vi "Extract Data.vi"(6 "Default body text":T1 {"Body Text Spec"."Alignment" items=["left", "center", "right"]}, 7 "Type":enum16{"VI", "Library"}(ring), 8 "error in":errorcluster, 11 "Value":variant) -> (0 "error out":errorcluster, 3 "Data":T4={"Text Visible?"=FALSE, "Text Opacity"=0, "Templ Visible?"=FALSE, "Templ Opacity"=0, "Relative Path from 1 to 2"=path "", "Image"=bytes[0], "All User Layers"=[], "Body Text"={"Line 1 text"="", "Line 2 text"="", "Line 3 text"="", "Line 4 text"="", "Line 1 color"=0, "Line 2 color"=0, "Line 3 color"=0, "Line 4 color"=0, "Body Text Spec"={"Font"="", "Alignment"=0, "Size"=3}, "Center text vertically"=FALSE, "Capitalize Text"=FALSE}} {"Body Text"."Body Text Spec"."Alignment" items=["left", "center", "right"]})   [LabVIEW 2012, in "lv_icon.lvlib"]
doc: "Extract the binary data of a LabVIEW Icon."
uses:
  <vilib>/LabVIEW Icon API/lv_icon/lv_icon.lvlib
  <vilib>/LabVIEW Icon API/lv_icon/Controls/LabVIEW Icon Stored Information.ctl
  <vilib>/LabVIEW Icon API/lv_icon/Classes/Layer/Layer.lvclass
  <vilib>/LabVIEW Icon API/lv_icon/Controls/BodyText.ctl
  <vilib>/LabVIEW Icon API/lv_icon/Controls/Font.ctl
  <vilib>/LabVIEW Icon API/lv_icon/Controls/Alignment.ctl
  <vilib>/picture/picture.llb/imagedata.ctl
  <vilib>/LabVIEW Icon API/lv_icon/Controls/LayerType.ctl
  <vilib>/LabVIEW Icon API/lv_icon/Classes/Load_Unload/Load & Unload.lvclass
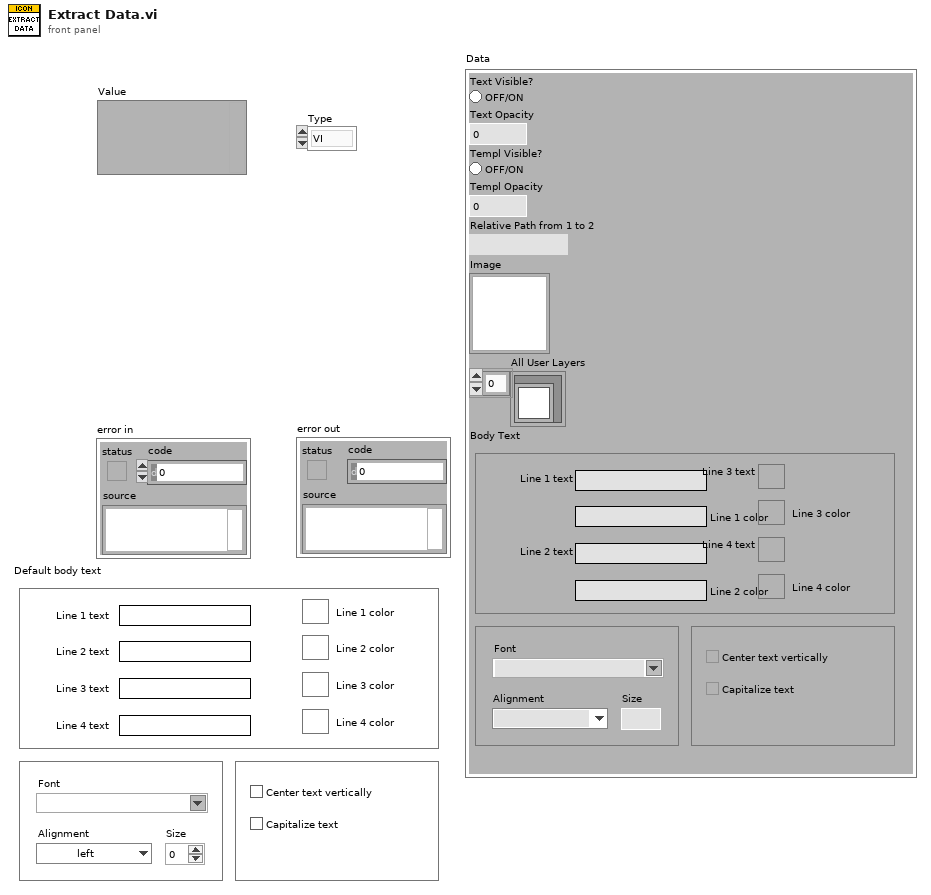
[diagram p1: front panel]
types:
  T1 = typedef "BodyText.ctl" = cluster{"Line 1 text":string, "Line 2 text":string, "Line 3 text":string, "Line 4 text":string, "Line 1 color":u32, "Line 2 color":u32, "Line 3 color":u32, "Line 4 color":u32, "Body Text Spec":cluster{"Font":T2, "Alignment":T3, "Size":u8}, "Center text vertically":bool, "Capitalize Text":bool}
  T2 = typedef "Font.ctl" = string
  T3 = typedef "Alignment.ctl" = u16
  T4 = typedef "LabVIEW Icon Stored Information.ctl" = cluster{"Text Visible?":bool, "Text Opacity":u8, "Templ Visible?":bool, "Templ Opacity":u8, "Relative Path from 1 to 2":path, "Image":picture, "All User Layers":refnum<class "Layer.lvclass">[], "Body Text":T1}
  T5 = typedef "imagedata.ctl" = cluster{"image type":i32, "image depth":i32, "image":u8[], "mask":u8[], "colors":u32[], "Rectangle":cluster{"left":i16, "top":i16, "right":i16, "bottom":i16}}
  T6 = cluster{string, "image data":T5, "image data":T5}
  T7 = typedef "LayerType.ctl" = enum16{"Graphic", "Text", "Tool", "Graphic Drop"}
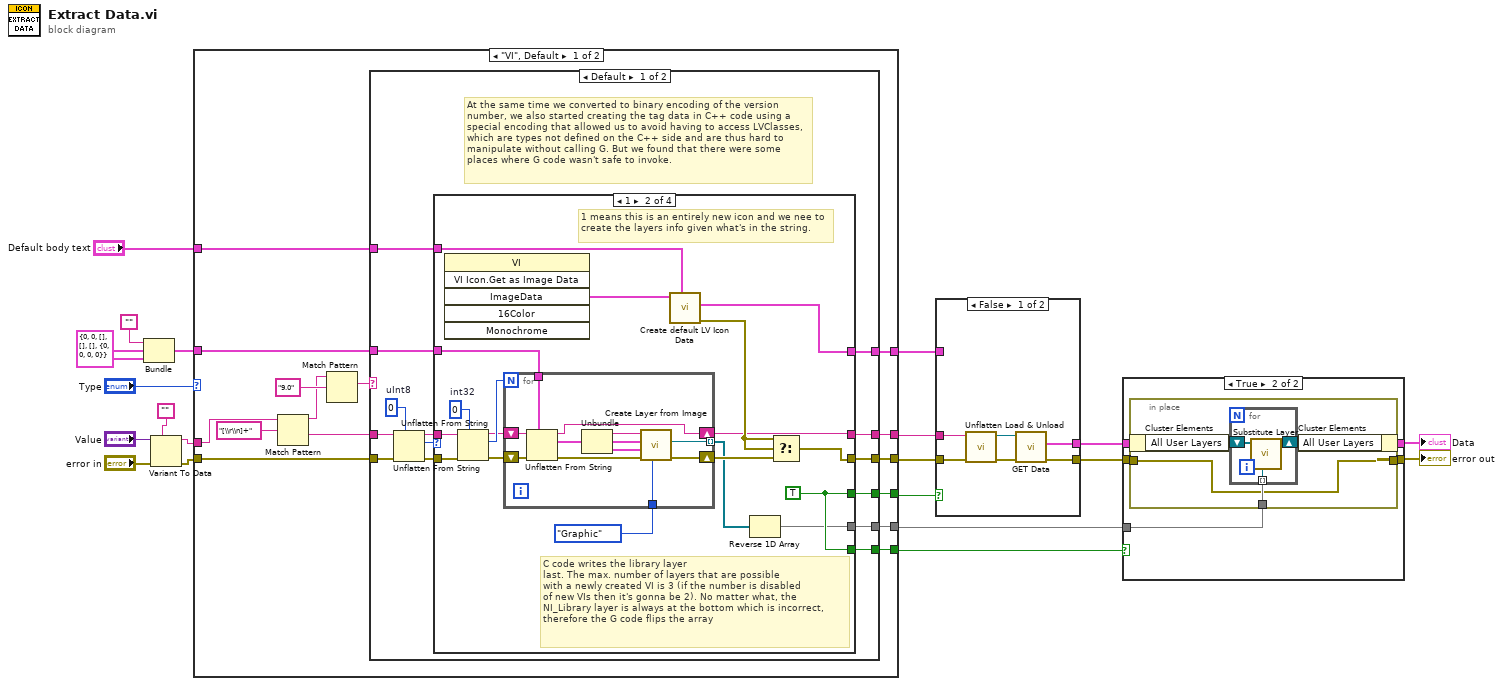
[diagram p0: block diagram]
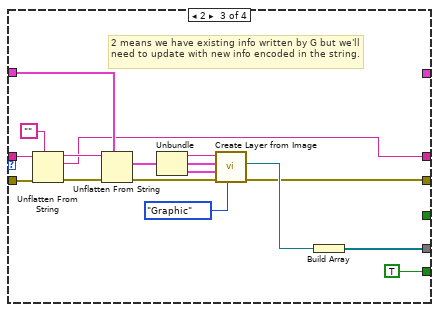
[diagram p5: hidden frame]
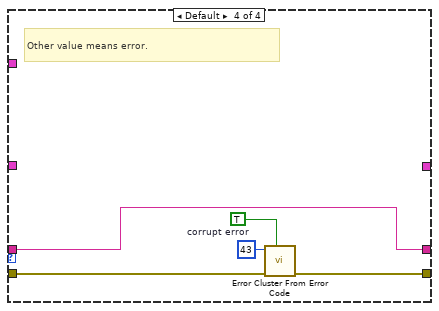
[diagram p6: hidden frame]
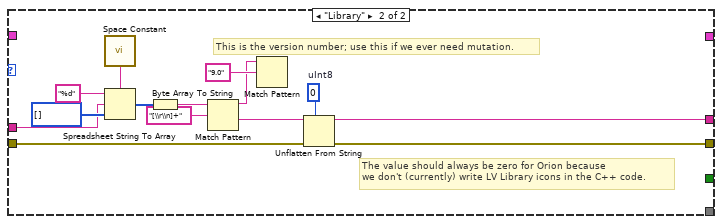
[diagram p8: hidden frame]
diagram:
  w8 = T5 {"image type"=0, "image depth"=0, "image"=[], "mask"=[], "colors"=[], "Rectangle"={"left"=0, "top"=0, "right"=0, "bottom"=0}} ("image data")
  n1 = Bundle("", "image data"=w8, "image data"=w8) -> (w9:T6)  [unwired: 1 in]
  n2 = Variant To Data(error in="error in", type="", Variant="Value") -> (data=w16:string, error out=w14:errorcluster)
  n3 = case shown="\"VI\", Default" "Type" {
    tunnel: w16 -> [w25 w115]
    tunnel: [w33 w106] -> w15
    tunnel: w14 -> [w32 w108]
    tunnel: [w31 w107] -> w13
    tunnel: [w30 _] -> w12
    tunnel: [w29 _] -> w11
    tunnel: w9 -> [w28 _]
    tunnel: [w27 _] -> w2
    tunnel: [w26 _] -> w7
    tunnel: "Default body text" -> [w21 _]
    frame "VI", Default {
      n4 = Match Pattern(string=w25, regular expression="[\\r\\n]+") -> (before substring=w24:string, after substring=w23:string)  [unwired: 1 in, 2 out]
      n5 = Match Pattern(string=w24, regular expression="9.0") -> (match substring=w34:string)  [unwired: 4 out]
      n6 = case shown="Default" w34 {
        tunnel: [w44 w105] -> w33
        tunnel: w23 -> [w49 w105]
        tunnel: w32 -> [w48 w104]
        tunnel: [w43 w104] -> w31
        tunnel: [w41 _] -> w30
        tunnel: [w40 _] -> w29
        tunnel: w28 -> [w39 _]
        tunnel: [w38 _] -> w27
        tunnel: [w37 _] -> w26
        tunnel: w21 -> [w36 _]
        frame Default {
          w47 = u8 0  # uInt8
          # "At the same time we converted to binary encoding of the version number, we also started creating the tag data in C++ code using a special encoding that allowed us to avoid having to access LVClasses, which are types not defined on the C++ side and are thus hard to manipulate without calling G. But we found that there were some places where G code wasn't safe to invoke."
          n7 = Unflatten From String(type=w47, binary string=w49, error in (no error)=w48) -> (rest of the binary string=w45:string, value=w46:u8, error out=w42:errorcluster)  [unwired: 2 out]
          n8 = case shown="1" w46 {
            tunnel: w45 -> [w51 w67 w97 w99]
            tunnel: [w51 w58 w87 w99] -> w44
            tunnel: [w50 w59 w85 w101] -> w43
            tunnel: w42 -> [w50 w68 w98 w102]
            tunnel: [_ w55 _ _] -> w41
            tunnel: [_ w56 _ _] -> w40
            tunnel: w39 -> [_ w62 w94 _]
            tunnel: [_ w53 w82 _] -> w38
            tunnel: [_ w55 TRUE _] -> w37
            tunnel: w36 -> [_ w52 _ _]
            frame 0 {
              # "Zero means this string was encoded in G code\nand the rest of string is just a flattened .lvclass,\nso pass it through."
            }
            frame 1 {
              w66 = 0  # int32
              w55 = TRUE
              # "C code writes the library layer\nlast. The max. number of layers that are possible\nwith a newly created VI is 3 (if the number is disabled\nof new VIs then it's gonna be 2). No matter what, the\nNI_Library layer is always at the bottom which is incorrect,\ntherefore the G code flips the array"
              # "1 means this is an entirely new icon and we nee to create the layers info given what's in the string."
              n9 = invoke class="VI" method="VI Icon.Get as Image Data"() -> ("ImageData"=w69:T5)  [unwired: 6 in, 5 out]
              n10 = Unflatten From String(type=w66, binary string=w67, error in (no error)=w68) -> (rest of the binary string=w64:string, value=w65:i32, error out=w63:errorcluster)  [unwired: 2 out]
              n11 = for {
                N: w65 -> [_]
                tunnel: w62 -> [w81]
                shift-right: [w75] -> w60
                shift-left: w63 -> [w79]
                shift-right: [w78] -> w58
                shift-left: w64 -> [w80]
                tunnel: [w74] -> w54 mode=indexing
                tunnel: LayerType."Graphic" ("Layer type") -> [w70]
                n12 = Unflatten From String(type=w81, binary string=w80, error in (no error)=w79) -> (rest of the binary string=w78:string, value=w77:T6, error out=w76:errorcluster)  [unwired: 2 out]
                n13 = Unbundle(w77) -> (w73:string, "image data"=w72:T5, "image data"=w71:T5)
                n14 = call <vilib>:"Create Layer from Image.vi"("Layer type"=w70, "error in"=w76, "Monochrome Data in"=w71, "Color Data In"=w72, "LayerName"=w73) -> ("error out"=w75:errorcluster, "Layer.lvclass out"=w74:refnum<class "Layer.lvclass">)  [unwired: 5 in]
              }
              n15 = call <vilib>:"Create default LV Icon Data.vi"("Body Text"=w52, "Pic Data in"=w69) -> ("error out"=w61:errorcluster, "VI Icon Data out"=w56:T4)  [unwired: 2 in, 6 out]
              n16 = Reverse 1D Array(array=w54) -> (reversed array=w53:refnum<class "Layer.lvclass">[])
              n17 = Select(t=w61, s=w61, f=w60) -> (s? t:f=w59:errorcluster)
            }
            frame 2 {
              # "2 means we have existing info written by G but we'll need to update with new info encoded in the string."
              n18 = Unflatten From String(type="", binary string=w97, error in (no error)=w98) -> (rest of the binary string=w96:string, value=w87:string, error out=w95:errorcluster)  [unwired: 2 out]
              n19 = Unflatten From String(type=w94, binary string=w96, error in (no error)=w95) -> (value=w93:T6, error out=w92:errorcluster)  [unwired: 3 out]
              n20 = Unbundle(w93) -> (w91:string, "image data"=w90:T5, "image data"=w89:T5)
              n21 = call <vilib>:"Create Layer from Image.vi"("Layer type"=LayerType."Graphic", "error in"=w92, "Monochrome Data in"=w89, "Color Data In"=w90, "LayerName"=w91) -> ("error out"=w85:errorcluster, "Layer.lvclass out"=w86:refnum<class "Layer.lvclass">)  [unwired: 5 in]
              n22 = Build Array(w86) -> (w82:refnum<class "Layer.lvclass">[])
            }
            frame Default {
              w103 = 43  # corrupt error
              # "Other value means error."
              n23 = call <vilib>:"Error Cluster From Error Code.vi"("show call chain? (False)"=TRUE, "error in (no error)"=w102, "error code (0)"=w103) -> ("error out"=w101:errorcluster)  [unwired: 6 in]
            }
          }
        }
        frame "9.0" {
          # "This VI was written before we started using the binary\nencoding of the version number. That means it does NOT\nhave any special encodings of the Load&Unload.lvclass\nembedded in it. So just pass it through to the standard unflatten."
        }
      }
    }
    frame "Library" {
      w110 = u8 0  # uInt8
      # "This is the version number; use this if we ever need mutation."
      # "The value should always be zero for Orion because\nwe don't (currently) write LV Library icons in the C++ code."
      n24 = call <vilib>:"Space Constant.vi"() -> ("String"=w119:string)
      n25 = Spreadsheet String To Array(delimiter (Tab)=w119, format string="%d", spreadsheet string=w115, array type (2D Dbl)=u8[] [] ("unsigned byte array")) -> (array=w117:u8[])
      n26 = Byte Array To String(unsigned byte array=w117) -> (string=w111:string)
      n27 = Match Pattern(string=w111, regular expression="[\\r\\n]+") -> (before substring=w113:string, after substring=w109:string)  [unwired: 1 in, 2 out]
      n28 = Match Pattern(string=w113, regular expression="9.0") -> ()  [unwired: 5 out]
      n29 = Unflatten From String(type=w110, binary string=w109, error in (no error)=w108) -> (rest of the binary string=w106:string, error out=w107:errorcluster)  [unwired: 3 out]
    }
  }
  n30 = case shown="False" w12 {
    tunnel: [w125 w126] -> w5
    tunnel: [w124 w127] -> w3
    tunnel: w15 -> [w121 _]
    tunnel: w13 -> [w123 w127]
    tunnel: w11 -> [_ w126]
    frame False {
      n31 = call <vilib>:"Unflatten Load & Unload.vi"("Error In"=w123, "String"=w121) -> ("Error Out"=w122:errorcluster, "Load & Unload.lvclass"=w120:refnum<class "Load & Unload.lvclass">)  [unwired: 8 in]
      n32 = call-dynamic "GET Data.vi"("error in (no error)"=w122, "Load & Unload.lvclass in"=w120) -> ("error out"=w124:errorcluster, "Data"=w125:T4)  [unwired: 8 out]
    }
    frame True {
    }
  }
  n33 = case shown="True" w7 {
    tunnel: [w129 w133] -> w6
    tunnel: w5 -> [w129 w134]
    tunnel: [w128 w131] -> w4
    tunnel: w3 -> [w128 w130]
    tunnel: w2 -> [_ w132]
    frame False {
    }
    frame True {
      n34 = in-place {
        in-place-border: w132 -> [w138]
        in-place-border: [w135] -> w131
        in-place-border: w130 -> [w135]
        n35 = in-place-cluster #1(w134) -> ("All User Layers"=w136:refnum<class "Layer.lvclass">[])
        n36 = for {
          tunnel: w138 -> [w141] mode=indexing
          shift-right: [w140] -> w137
          shift-left: w136 -> [w139]
          n37 = call <vilib>:"Substitute Layer.vi"("Substitute Layer"=w141, "All User Layers in"=w139) -> ("All User Layers out"=w140:refnum<class "Layer.lvclass">[])  [unwired: 9 in]
        }
        n38 = in-place-cluster #1("All User Layers"=w137) -> (w133:T4)
      }
    }
  }
  "Data" <- w6
  "error out" <- w4
